vi "Чтение КС (SubVI).vi"(10 "КС для обработки":bool[](array[boolean]), 11 "Адрес ОУ (0-31)":u8=8) -> (0 "Подадрес":u32, 1 "Кол-во СД":u32, 2 "Передача данных на ОУ?":bool, 3 "КС верно?":bool)   [LabVIEW 2015]
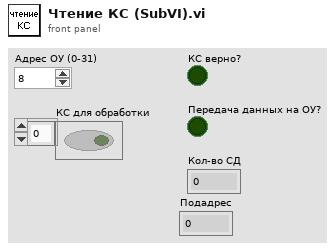
[diagram p1: front panel]
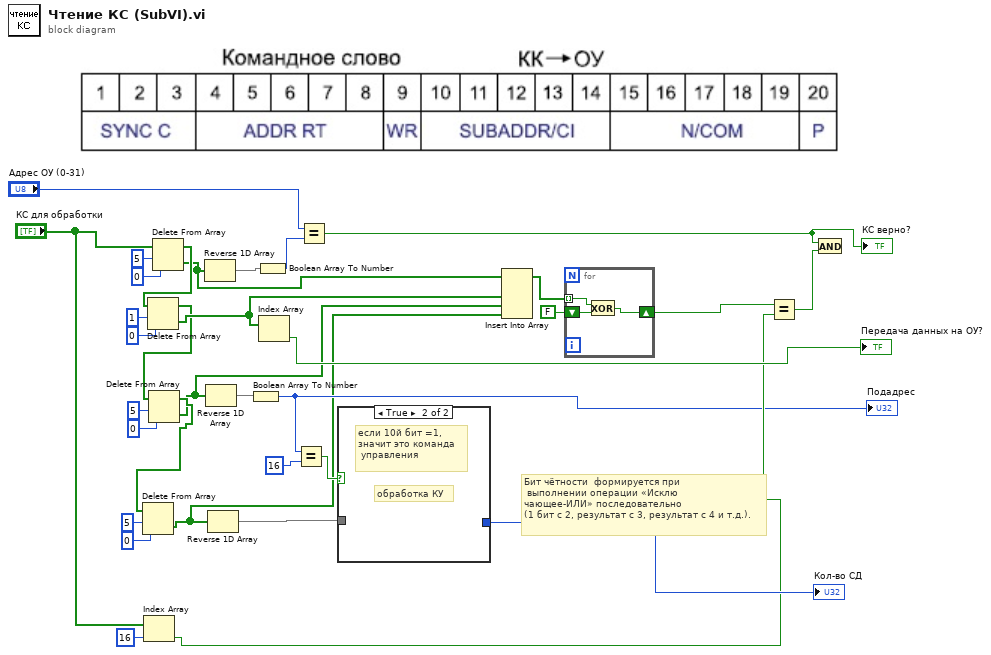
[diagram p0: block diagram]
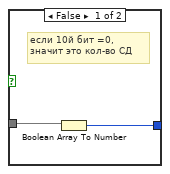
[diagram p2: hidden frame]
diagram:
  # "Бит чётности  формируется при\n выполнении операции «Исклю\nчающее-ИЛИ» последовательно \n(1 бит с 2, результат с 3, результат с 4 и т.д.)."
  n1 = Index Array(array="КС для обработки", index=16) -> (element=w16:bool)
  n2 = Delete From Array(array="КС для обработки", length=5, index=0) -> (deleted portion=w3:bool[], array with subset deleted=w30:bool[])
  n3 = Delete From Array(array=w30, length=1, index=0) -> (deleted portion=w13:bool[], array with subset deleted=w10:bool[])
  n4 = Delete From Array(array=w10, length=5, index=0) -> (deleted portion=w5:bool[], array with subset deleted=w8:bool[])
  n5 = Delete From Array(array=w8, length=5, index=0) -> (deleted portion=w4:bool[])  [unwired: 1 out]
  n6 = Reverse 1D Array(array=w3) -> (reversed array=w14:bool[])
  n7 = Reverse 1D Array(array=w5) -> (reversed array=w9:bool[])
  n8 = Reverse 1D Array(array=w4) -> (reversed array=w6:bool[])
  n9 = Boolean Array To Number(Boolean array=w9) -> (number=w7:u32)
  "Подадрес" <- w7
  n10 = Boolean Array To Number(Boolean array=w14) -> (number=w23:u32)
  n11 = Index Array(array=w13) -> (element=→"Передача данных на ОУ?":bool)  [unwired: 1 in]
  n12 = Equal?(x=w7, y=16) -> (x = y?=w28:bool)
  n13 = Equal?(x="Адрес ОУ (0-31)", y=w23) -> (x = y?=w1:bool)
  "КС верно?" <- w1
  n14 = case shown="True" w28 {
    tunnel: [w35 _] -> w29
    tunnel: w6 -> [w34 _]
    frame False {
      # "если 10й бит =0,\nзначит это кол-во СД"
      n15 = Boolean Array To Number(Boolean array=w34) -> (number=w35:u32)
    }
    frame True {
      # "если 10й бит =1,\nзначит это команда\n управления"
      # "обработка КУ"
    }
  }
  "Кол-во СД" <- w29
  n16 = Insert Into Array(array=w3, new element #1=w13, new element #2=w5, new element #3=w4) -> (w21:bool[])  [unwired: 1 in]
  n17 = for {
    tunnel: w21 -> [w38] mode=indexing
    shift-right: [w37] -> w17
    shift-left: FALSE -> [w36]
    n18 = Exclusive Or(1:w36, 2:w38) -> (0:w37:bool)
  }
  n19 = Equal?(x=w17, y=w16) -> (x = y?=w15:bool)
  n20 = And(x=w1, y=w15) -> ()  [unwired: 1 out]
